vi "TCP IP Parse BipolarPowerMilliwatts.vi"(11 "JSON in":string) -> (2 "Bipolar Power (xx.x)":string, 3 "JSON out":string)   [LabVIEW 2015]
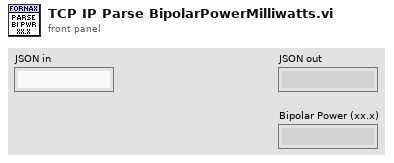
[diagram p1: front panel]
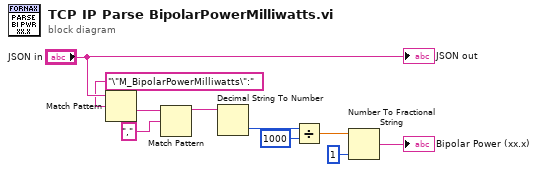
[diagram p0: block diagram]
diagram:
  n1 = Match Pattern(string="JSON in", regular expression="\"M_BipolarPowerMilliwatts\":") -> (after substring=w2:string)  [unwired: 1 in, 3 out]
  n2 = Match Pattern(string=w2, regular expression=",") -> (before substring=w5:string)  [unwired: 1 in, 3 out]
  n3 = Decimal String To Number(string=w5) -> (number=w6:i32)  [unwired: 2 in, 1 out]
  n4 = Divide(x=w6, y=1000) -> (x/y=w9:dbl)
  n5 = Number To Fractional String(number=w9, precision (6)=i16 1) -> (F-format string=→"Bipolar Power (xx.x)":string)  [unwired: 2 in]
  "JSON out" <- "JSON in"
